vi "Acquire.vi"(8 "error in (no error)":errorcluster, 11 "Image":refnum<data-value>) -> (0 "error out":errorcluster, 3 "Mapped Memory Access Image Greyscale":refnum<data-value>)   [LabVIEW 2020, in "g_ar_toolkit.image.lvlib" / "Mapped Memory Access Image Greyscale.lvclass"]
uses:
  Mapped Memory Access Image Greyscale.lvclass
  Mapped Memory Access Image Greyscale.lvclass/Mapped Memory Access Image Greyscale.ctl
  09df33ca-1321-4267-b217-b72c9be7f03b.vi
  <vilib>/Utility/error.llb/Error Cluster From Error Code.vi
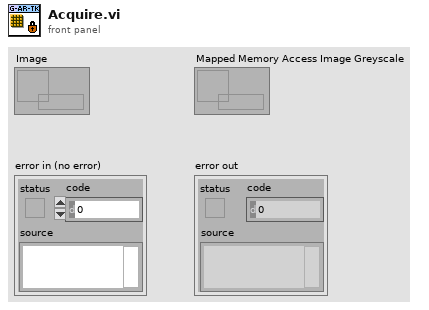
[diagram p1: front panel]
types:
  T1 = typedef "g_ar_toolkit.image.lvlib/Raw Memory Information.ctl" = cluster{"Memory Address":u64, "Dimension 0":T2, "Dimension 1":T2}
  T2 = typedef "g_ar_toolkit.image.lvlib/Raw Memory Information Dimension.ctl" = cluster{"Size":u16, "Stride":u32}
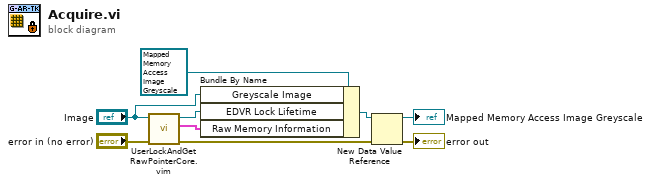
[diagram p0: block diagram]
diagram:
  n1 = call "UserLockAndGetRawPointerCore.vim"("error in (no error)"="error in (no error)", "Image"="Image") -> ("error out"=w4:errorcluster, "Raw Memory Information"=w1:T1, "EDVR Lock Lifetime"=w3:refnum<data-value>)  [unwired: 7 in]
  n2 = Bundle By Name(cluster=refnum<class "Mapped Memory Access Image Greyscale.lvclass"> refnum ("Locked Image ARGB in"), "Greyscale Image"="Image", "EDVR Lock Lifetime"=w3, "Raw Memory Information"=w1) -> (w8:refnum<class "Mapped Memory Access Image Greyscale.lvclass">)
  n3 = New Data Value Reference(data value=w8, error in=w4) -> (data value reference=→"Mapped Memory Access Image Greyscale":refnum<data-value>, error out=→"error out":errorcluster)
